vi "Andor_to_xml.vi"(8 "error in":errorcluster, 11 "Andor settings":T1) -> (0 "error out":errorcluster, 3 "settings string":string)   [LabVIEW 2013]
doc: "Saves HSDIO settings in the format:\n\n<EnableHSDIOPulses>%b</EnableHSDIOPulses>\n<ResourceName>%s</ResourceName>\n<ClockRate>%f</ClockRate>\n<unitsPerSecond>%f</unitsPerSecond>\n<HardwareAlignmentQuantum units=\"samples\">%u</HardwareAlignmentQuantum>\n<ArrayOfScriptTriggers columns=\"id, source, type, edge, level\">\n<trigger>%s\\t%s\\t%s\\t%s\\t%s</trigger>\n</ArrayOfScriptTriggers>\n<ChannelsControl columns=\"Description, Active?, Idle State\">\n<channel>%s</channel>\n</ChannelsControl>\n<PulseGenerationScript>%s</PulseGenerationScript>\n<DirectoryToLookForWaveformFiles>%s</DirectoryToLookForWaveformFiles>\n<StartTrigger.WaitForStartTrigger>%b</StartTrigger.WaitForStartTrigger>\n<StartTrigger.source>%s</StartTrigger.source>\n<StartTrigger.edge>%s</StartTrigger.edge>\n\nMTL 2013 Jan 1"
uses:
  Camera/Andor/Andor_settings.ctl
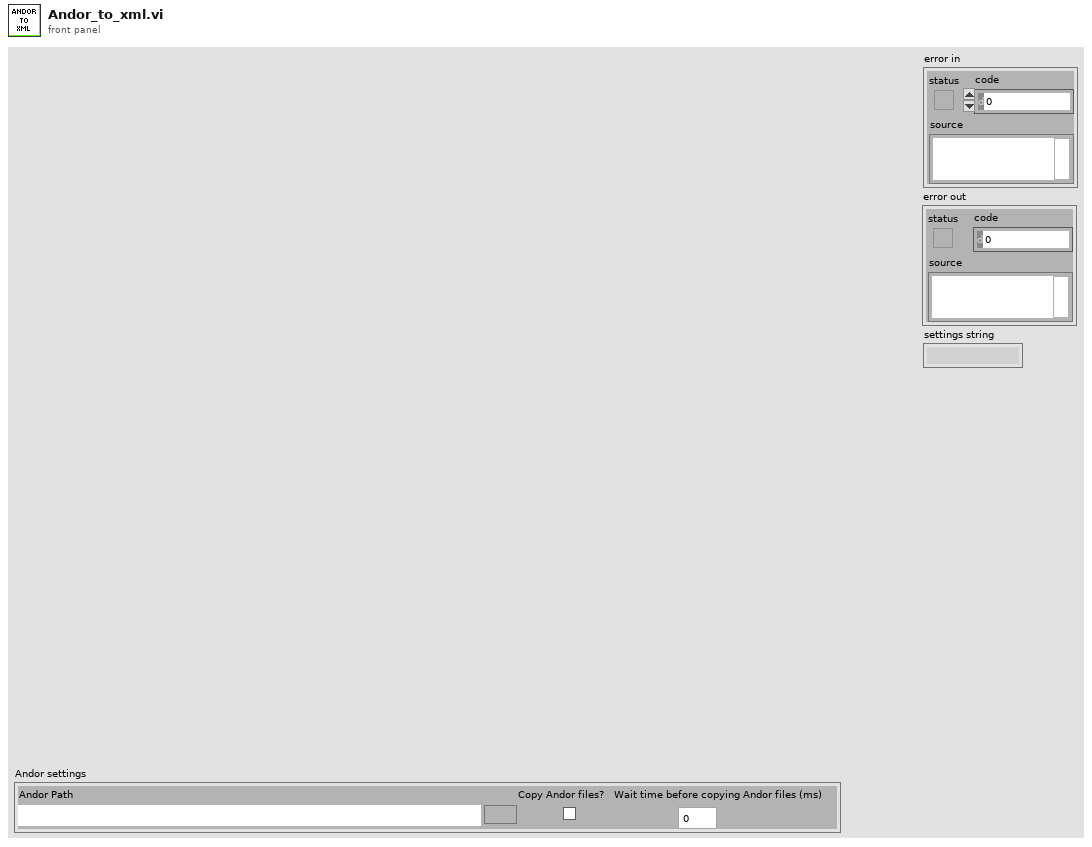
[diagram p1: front panel]
types:
  T1 = typedef "Andor_settings.ctl" = cluster{"Andor Path":path, "Copy any Andor files":bool, "Wait time before copying Andor files (ms)":u16}
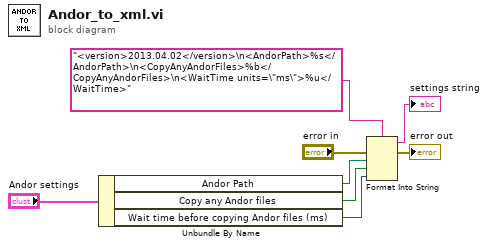
[diagram p0: block diagram]
diagram:
  n1 = Unbundle By Name("Andor settings") -> ("Andor Path"=w4:path, "Copy any Andor files"=w3:bool, "Wait time before copying Andor files (ms)"=w2:u16)
  n2 = Format Into String(format string="<version>2013.04.02</version>\n<AndorPath>%s</AndorPath>\n<CopyAnyAndorFiles>%b</CopyAnyAndorFiles>\n<WaitTime units=\"ms\">%u</WaitTime>", error in="error in", w4, w3, w2) -> (resulting string=→"settings string":string, error out=→"error out":errorcluster)  [unwired: 1 in]
